vi "Exercises_4-4.vi"(1 "Power":bool) -> ()   [LabVIEW 2014]
doc: "This VI simulates measuring a temperature using the temperature sensor on the DAQ Signal Accessory.\n\nIf you have a DAQ board or a DAQ Signal Accessory, then use the Thermometer VI instead."
panel:
  out "Temperature History":dbl(graph)
  # "ON\n\nOFF"
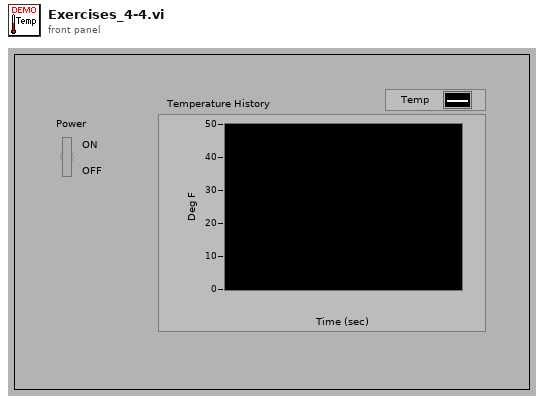
[diagram p1: front panel]
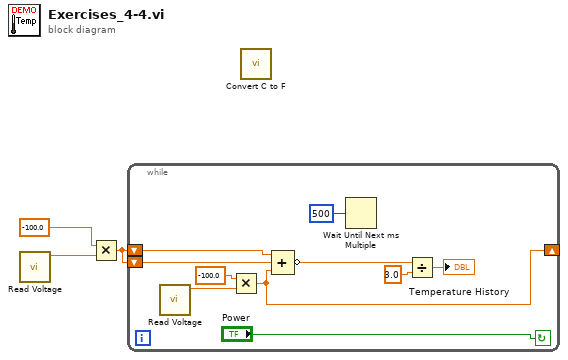
[diagram p0: block diagram]
diagram:
  n1 = call "Read Voltage.vi"() -> ("voltaje"=w2:dbl)  [unwired: 6 in, 1 out]
  n2 = Multiply(x=-100.0, y=w2) -> (x*y=w1:dbl)
  n3 = while {
    shift-right: [w4] -> _
    shift-left: w1 -> [w9]
    shift-left: w1 -> [w8]
    stop <- "Power" continue-if-true
    n4 = call "Read Voltage.vi"() -> ("voltaje"=w5:dbl)  [unwired: 6 in, 1 out]
    n5 = Multiply(x=-100.0, y=w5) -> (x*y=w4:dbl)
    n6 = Compound Arithmetic op=ADD(w9, w8, w4) -> (invert w12:dbl)
    n7 = Wait Until Next ms Multiple(millisecond multiple=500) -> ()  [unwired: 1 out]
    n8 = Divide(x=w12, y=3.0) -> (x/y=→"Temperature History":dbl)
  }
  n9 = call "Convert C to F.vi"() -> ()  [unwired: 1 in, 1 out]
